vi "Post-Build Action.vi"(5 "Files Generated by Build":path[](array[path]), 6 "Top Level/Always Included VIs":path[](array[path]), 7 "Destination Path":path, 8 "error in (no error)":errorcluster, 9 "Target Name":string, 10 "Build Specification Name":string, 11 "Project Path":path) -> (0 "error out":errorcluster)   [LabVIEW 2020]
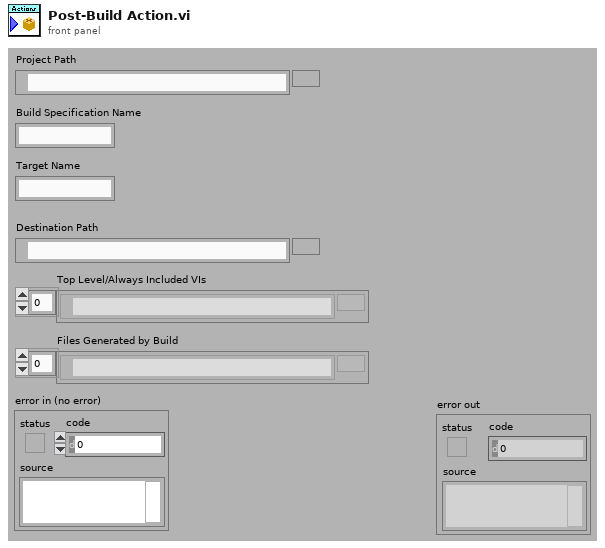
[diagram p1: front panel]
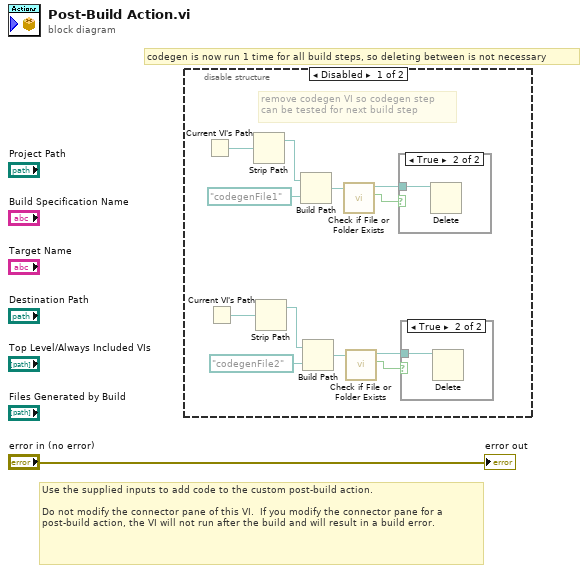
[diagram p0: block diagram]
diagram:
  # "codegen is now run 1 time for all build steps, so deleting between is not necessary"
  # "Use the supplied inputs to add code to the custom post-build action.\n\nDo not modify the connector pane of this VI.  If you modify the connector pane for a post-build action, the VI will not run after the build and will result in a build error."
  n1 = disable-structure shown="Disabled" {
    frame Disabled {
      # "remove codegen VI so codegen step \ncan be tested for next build step"
      n2 = Current VI's Path() -> (path=w13:path)
      n3 = Current VI's Path() -> (path=w2:path)
      n4 = Strip Path(path=w13) -> (stripped path=w12:path)  [unwired: 1 out]
      n5 = Strip Path(path=w2) -> (stripped path=w3:path)  [unwired: 1 out]
      n6 = Build Path(base path=w12, name or relative path=path "codegenFile1") -> (appended path=w10:path)
      n7 = Build Path(base path=w3, name or relative path=path "codegenFile2") -> (appended path=w5:path)
      n8 = call <vilib>:"Check if File or Folder Exists.vi"("path"=w10) -> ("file or folder exists?"=w9:bool, "dup path"=w8:path)  [unwired: 8 in, 1 out]
      n9 = call <vilib>:"Check if File or Folder Exists.vi"("path"=w5) -> ("file or folder exists?"=w6:bool, "dup path"=w7:path)  [unwired: 8 in, 1 out]
      n10 = case shown="True" w9 {
        tunnel: w8 -> [_ w15]
        frame False {
        }
        frame True {
          n11 = Delete(path (use dialog)=w15) -> ()  [unwired: 4 in, 3 out]
        }
      }
      n12 = case shown="True" w6 {
        tunnel: w7 -> [_ w14]
        frame False {
        }
        frame True {
          n13 = Delete(path (use dialog)=w14) -> ()  [unwired: 4 in, 3 out]
        }
      }
    }
    frame Enabled {
    }
  }
  "error out" <- "error in (no error)"
